vi "search_cv.vi"(6 "regex":string, 8 "Sort Type":enum16{"Fuzzy", "Regex"}(ring), 9 "Array in":string[][](array[string]), 10 "compare threshold":dbl=0.5 format="%#_13g", 11 "search value":string) -> (3 "search results":string[][](array[string]))   [LabVIEW 2024, in "CLZ_to_ComicVine.lvlib" / "CLZ Comics.lvclass"]
uses:
  CLZ Comics.lvclass
  CLZ Comics.lvclass/CLZ Comics.ctl
  <userlib>/_OpenG.lib/string/string.llb/openg_string.lvlib
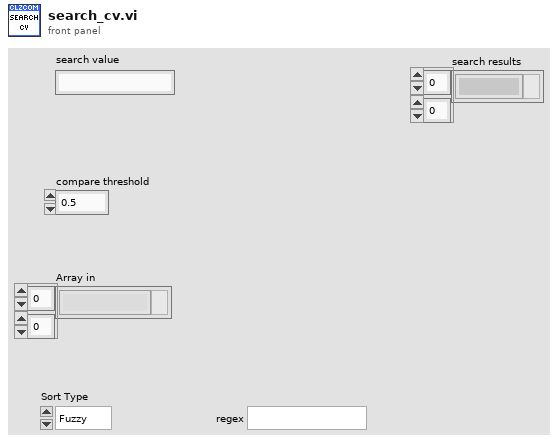
[diagram p1: front panel]
types:
  T1 = cluster{dbl, "name":string, "Array in":string[]}[]
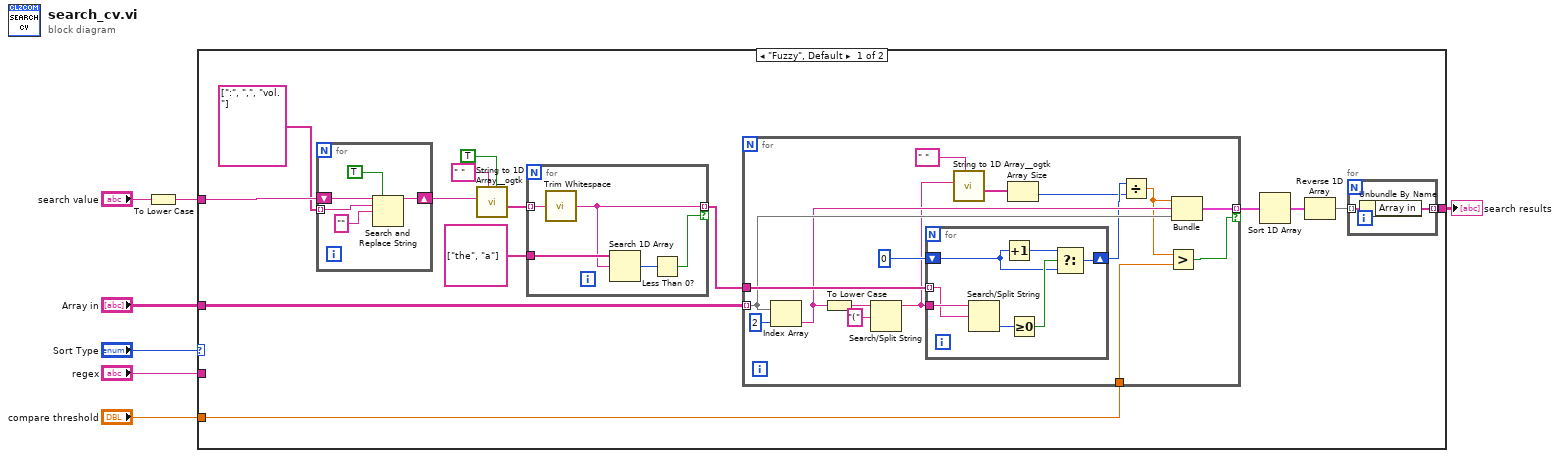
[diagram p0: block diagram]
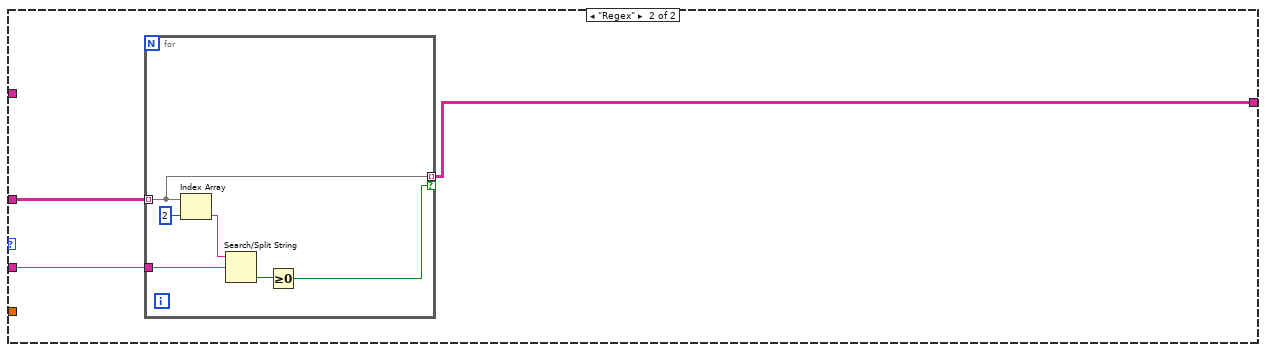
[diagram p2: hidden frame]
diagram:
  n1 = To Lower Case(string="search value") -> (all lower case string=w4:string)
  n2 = case shown="\"Fuzzy\", Default" "Sort Type" {
    tunnel: [w14 w57] -> w6
    tunnel: "Array in" -> [w13 w59]
    tunnel: w4 -> [w12 _]
    tunnel: "compare threshold" -> [w8 _]
    tunnel: "regex" -> [_ w58]
    frame "Fuzzy", Default {
      n3 = for {
        shift-right: [w22] -> w10
        shift-left: w12 -> [w26]
        tunnel: string[] [":", ",", "vol."] -> [w25] mode=indexing
        n4 = Search and Replace String(replace all?=TRUE ("replace all? (F)"), input string=w26, search string=w25, replace string="" ("replace string (\"\")")) -> (result string=w22:string)  [unwired: 4 in, 3 out]
      }
      n5 = call <userlib>:"String to 1D Array__ogtk.vi"("ignore duplicate delimiters? (F=No)"=TRUE, "delimiter (Tab)"=" ", "string"=w10) -> ("Array of Strings"=w20:string[])  [unwired: 8 in]
      n6 = for {
        tunnel: w20 -> [w32] mode=indexing
        tunnel: string[] ["the", "a"] -> [w33]
        tunnel: [w29] -> w18 mode=indexing if=w30
        n7 = call <vilib>:"Trim Whitespace.vi"("string"=w32) -> ("trimmed string"=w29:string)  [unwired: 1 in]
        n8 = Search 1D Array(1D array=w33, element=w29) -> (index of element=w31:i32)  [unwired: 1 in]
        n9 = Less Than 0?(x=w31) -> (x < 0?=w30:bool)
      }
      n10 = for {
        tunnel: w18 -> [w49]
        tunnel: [w47] -> w17 mode=indexing if=w41
        tunnel: w13 -> [w46] mode=indexing
        tunnel: w8 -> [w34]
        n11 = Index Array(array=w46, index=2) -> (element=w44:string)
        n12 = To Lower Case(string=w44) -> (all lower case string=w40:string)
        n13 = Search/Split String(string=w40, search string/char (-)="(") -> (substring before match=w38:string)  [unwired: 1 in, 2 out]
        n14 = for {
          tunnel: w49 -> [w55] mode=indexing
          tunnel: w38 -> [w56]
          shift-right: [w50] -> w43
          shift-left: 0 -> [w52]
          n15 = Search/Split String(string=w56, search string/char (-)=w55) -> (offset of match=w54:i32)  [unwired: 1 in, 2 out]
          n16 = Increment(x=w52) -> (x+1=w51:i32)
          n17 = Greater Or Equal To 0?(x=w54) -> (x >= 0?=w53:bool)
          n18 = Select(t=w51, s=w53, f=w52) -> (s? t:f=w50:i32)
        }
        n19 = call <userlib>:"String to 1D Array__ogtk.vi"("delimiter (Tab)"=" ", "string"=w38) -> ("Array of Strings"=w36:string[])  [unwired: 9 in]
        n20 = Array Size(array=w36) -> (size(s)=w35:i32)
        n21 = Divide(x=w43, y=w35) -> (x/y=w42:dbl)
        n22 = Greater?(x=w42, y=w34) -> (0:w41:bool)
        n23 = Bundle(w42, "name"=w44, "Array in"=w46) -> (w47:cluster{dbl, "name":string, "Array in":string[]})  [unwired: 1 in]
      }
      n24 = Sort 1D Array(array=w17) -> (sorted array=w16:T1)
      n25 = Reverse 1D Array(array=w16) -> (reversed array=w15:T1)
      n26 = for {
        tunnel: w15 -> [w28] mode=indexing
        tunnel: [w27] -> w14 mode=indexing
        n27 = Unbundle By Name(w28) -> ("Array in"=w27:string[])
      }
    }
    frame "Regex" {
      n28 = for {
        tunnel: w59 -> [w61] mode=indexing
        tunnel: w58 -> [w63]
        tunnel: [w61] -> w57 mode=indexing if=w60
        n29 = Index Array(array=w61, index=2) -> (element=w64:string)
        n30 = Search/Split String(string=w64, search string/char (-)=w63) -> (offset of match=w62:i32)  [unwired: 1 in, 2 out]
        n31 = Greater Or Equal To 0?(x=w62) -> (x >= 0?=w60:bool)
      }
    }
  }
  "search results" <- w6
